vi "ClearQuestionData_Paper1(SubVI).vi"(11 "Refnum in":T1) -> ()   [LabVIEW 2013]
uses:
  <vilib>/addons/database/Connection.llb/Conn ObjectReference.ctl
  <vilib>/addons/database/Connection.llb/DB Tools Open Connec (String).vi
  <vilib>/addons/database/NI_Database_API.lvlib
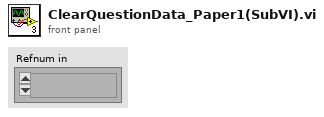
[diagram p1: front panel]
types:
  T1 = typedef "NI_Database_API.lvlib/Conn ObjectReference.ctl" = refnum<k1>
  T2 = cluster{string, string, string, string, string, string, string, string, string, string}
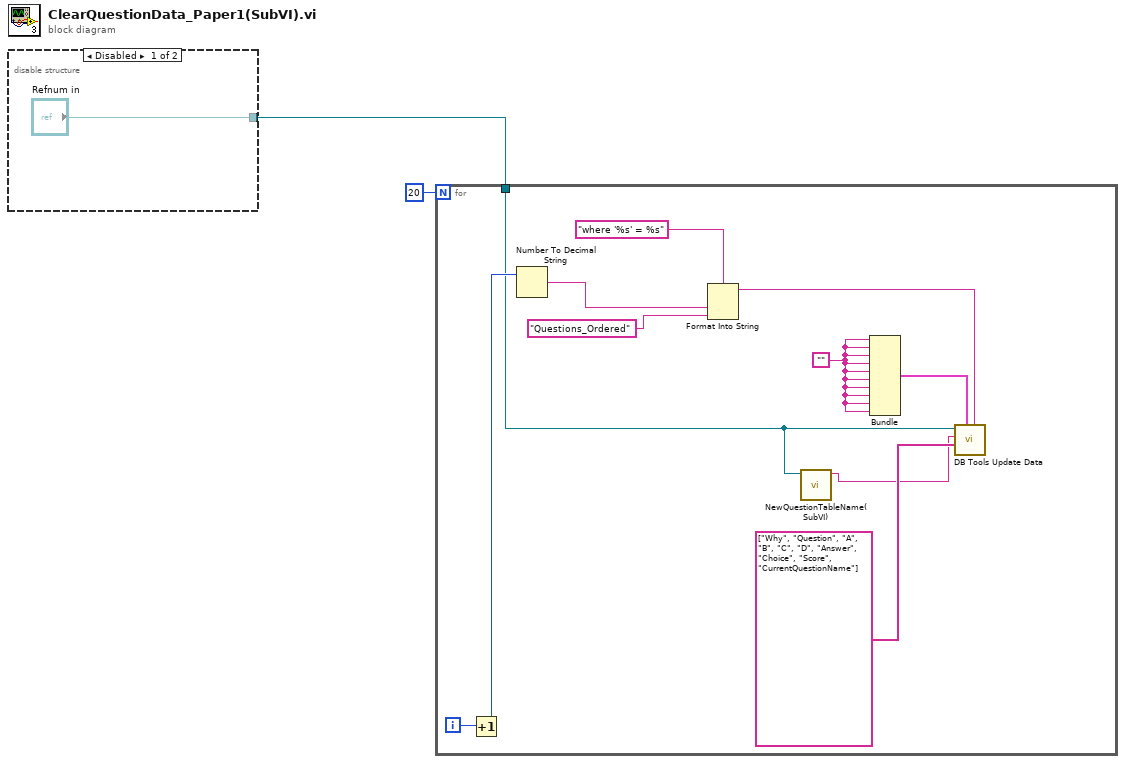
[diagram p0: block diagram]
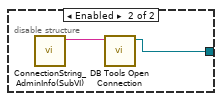
[diagram p2: hidden frame]
diagram:
  n1 = disable-structure shown="Disabled" {
    disable-tunnel: ["Refnum in" w4] -> w2
    frame Disabled {
    }
    frame Enabled {
      n2 = call "ConnectionString_AdminInfo(SubVI).vi"() -> ("ConnectionString"=w5:string)  [unwired: 11 in]
      n3 = call-poly <vilib>:"DB Tools Open Connection.vi"("connection information"=w5) -> ("connection reference"=w4:T1)  [unwired: 7 in, 1 out]
    }
  }
  n4 = for {
    N: 20 -> [_]
    tunnel: w2 -> [w7]
    i -> [w11]
    w6 = ""
    n5 = Increment(x=w11) -> (x+1=w10:i32)
    n6 = Number To Decimal String(number=w10) -> (decimal integer string=w12:string)  [unwired: 1 in]
    n7 = Format Into String(format string="where '%s' = %s", w12, "Questions_Ordered") -> (resulting string=w13:string)  [unwired: 2 in, 1 out]
    n8 = call "NewQuestionTableName(SubVI).vi"("connection reference"=w7) -> ("String"=w8:string)  [unwired: 9 in, 1 out]
    n9 = Bundle(w6, w6, w6, w6, w6, w6, w6, w6, w6, w6) -> (w9:T2)  [unwired: 1 in]
    n10 = call <vilib>:"DB Tools Update Data.vi"("condition"=w13, "data"=w9, "columns"=string[] ["Why", "Question", "A", "B", "C", "D", "Answer", "Choice", "Score", "CurrentQuestionName"], "table"=w8, "connection reference"=w7) -> ()  [unwired: 5 in, 2 out]
  }
